vi "BLED1112_app-discovery scan.vi"(0 "COM in":refnum<visa-resource-name>="COM8", 9 "Device List":refnum<vi>, 11 "LED ref":refnum<vi>) -> (4 "COM out":refnum<visa-resource-name>, 6 "BLED112 Dongle Info":string="Major: 1, Minor: 3, Patch: 2, Build: 122, LL ver: 3, Protocol ver: 1 and HW ver: 3  ", 8 "Device List":i32(listbox)=2, 10 "Scan success?":bool, 15 "error out":errorcluster caption="에러 출력")   [LabVIEW 2015]
panel:
  # "BLE Discovery"
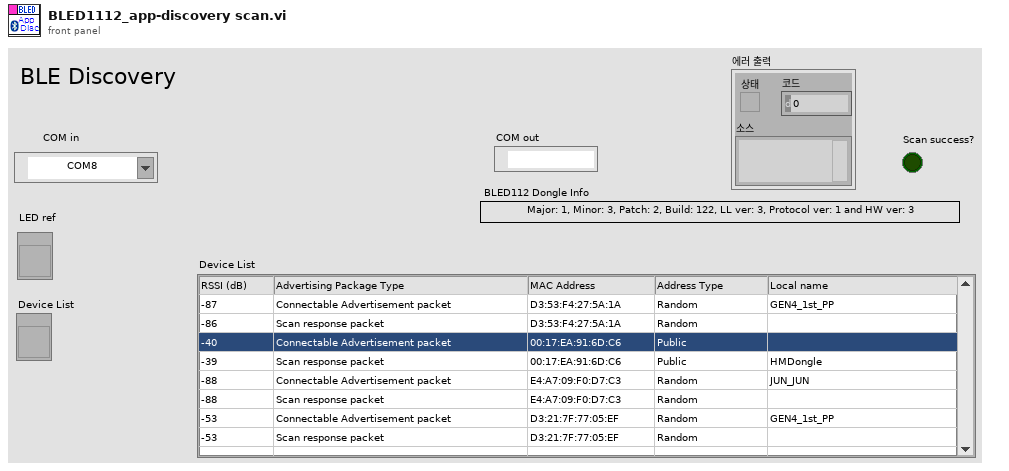
[diagram p1: front panel]
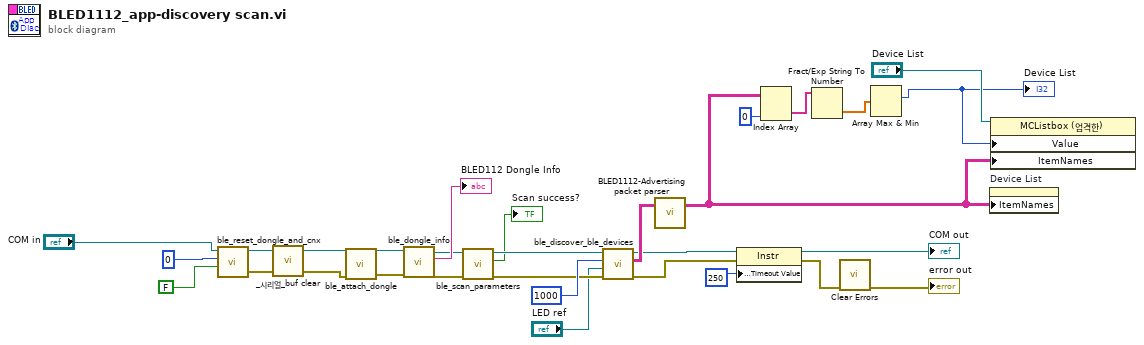
[diagram p0: block diagram]
diagram:
  n1 = call "ble_reset_dongle_and_cnx.vi"("Reset?"=FALSE, "wait time (100)"=u32 0, "COM Bluegiga in"="COM in") -> ("error out"=w11:errorcluster, "COM Bluegiga out"=w12:refnum<visa-resource-name>)  [unwired: 7 in]
  n2 = call "_시리얼_buf clear.vi"("에러 출력 2"=w11, "시리얼 포트"=w12) -> ("에러 출력"=w9:errorcluster, "시리얼 포트 2"=w10:refnum<visa-resource-name>)  [unwired: 2 in]
  n3 = call "ble_attach_dongle.vi"("error in (no error)"=w9, "COM Bluegiga in"=w10) -> ("error out"=w17:errorcluster, "COM Bluegiga out"=w18:refnum<visa-resource-name>)  [unwired: 8 in]
  n4 = call "ble_dongle_info.vi"("error in (no error)"=w17, "COM Bluegiga in"=w18) -> ("error out"=w27:errorcluster, "info"=→"BLED112 Dongle Info":string, "COM Bluegiga out"=w28:refnum<visa-resource-name>)  [unwired: 7 in]
  n5 = call "ble_scan_parameters.vi"("error in (no error)"=w27, "COM Bluegiga in"=w28) -> ("error out"=w25:errorcluster, "success?"=→"Scan success?":bool, "COM Bluegiga out"=w26:refnum<visa-resource-name>)  [unwired: 7 in]
  n6 = call "ble_discover_ble_devices.vi"("error in (no error)"=w25, "LED ref"="LED ref", "Scan Duration (10000ms)"=u32 1000, "COM Bluegiga in"=w26) -> ("error out"=w21:errorcluster, "Devices"=w23:string[][], "COM Bluegiga out"=w22:refnum<visa-resource-name>)  [unwired: 5 in]
  n7 = call "BLED1112-Advertising  packet parser.vi"("Advertising Data (in)"=w23) -> ("Advertising Data  (out)"=w2:string[][])  [unwired: 2 in]
  n8 = property class="Instr"(reference=w22, error in=w21, "General Settings:Timeout Value"=u32 250) -> (reference out=→"COM out":refnum<visa-resource-name>, error out=w20:errorcluster)
  n9 = Index Array(array=w2, index (col)=0 ("비활성화된 인덱스 (열)")) -> (element=w15:string[])  [unwired: 1 in]
  n10 = Fract/Exp String To Number(string=w15) -> (number=w14:dbl[])  [unwired: 3 in, 1 out]
  n11 = call <vilib>:"Clear Errors.vi"("error in (no error)"=w20) -> ("error out"=→"error out":errorcluster)  [unwired: 5 in, 1 out]
  n12 = Array Max & Min(array=w14) -> (max index (indices)=w3:i32)  [unwired: 3 out]
  "Device List" <- w3
  n13 = property on="Device List" class="MCListbox (엄격한)"("ItemNames"=w2) -> ()  [unwired: 2 in, 2 out]
  n14 = property class="MCListbox (엄격한)"(reference="Device List", "Value"=w3, "ItemNames"=w2) -> ()  [unwired: 1 in, 2 out]
